vi "NI Switch Init.vi"(8 "error in (no error)":errorcluster, 9 "topology name":T1="Configured Topology", 10 "resource name":refnum<k15>="PXI1Slot3_2_ivi", 11 "object in":refnum<class "NISwitch.lvclass">) -> (0 "error out":errorcluster, 3 "object out":refnum<class "NISwitch.lvclass">)   [LabVIEW 2023, in "HardwareAbstractionLayer_LVOOP.lvlib" / "NISwitch.lvclass"]
uses:
  NISwitch.lvclass
  <instrlib>/niSwitch/niSwitch.llb/niSwitch Topologies.ctl
  NISwitch.lvclass/NISwitch.ctl
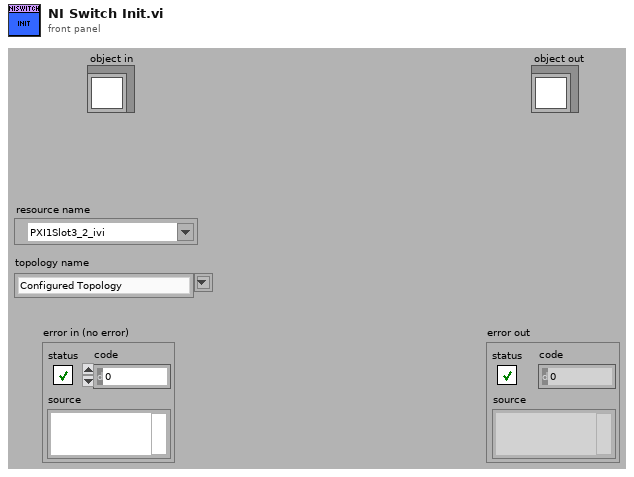
[diagram p1: front panel]
types:
  T1 = typedef "niSwitch Topologies.ctl" = string
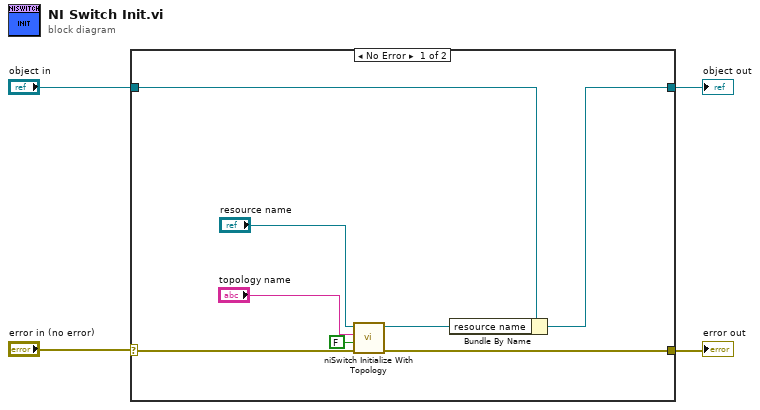
[diagram p0: block diagram]
diagram:
  n1 = case shown="No Error" "error in (no error)" {
    selector: "error in (no error)" -> [w10 w13]
    tunnel: "object in" -> [w12 w14]
    tunnel: [w11 w14] -> w3
    tunnel: [w9 w13] -> w1
    frame No Error {
      n2 = call <instrlib>:"niSwitch Initialize With Topology.vi"("error in (no error)"=w10, "reset device (boolean value)"=FALSE, "topology name"="topology name", "resource name"="resource name") -> ("error out"=w9:errorcluster, "instrument handle out"=w8:refnum<k15>)  [unwired: 6 in]
      n3 = Bundle By Name(cluster=w12, "resource name"=w8) -> (w11:refnum<class "NISwitch.lvclass">)
    }
    frame Error {
    }
  }
  "object out" <- w3
  "error out" <- w1
